vi "Convert_ERDs_ARG.vi"(0 "New Header?":bool, 2 "ERD Name":string[](array[string]), 5 "All_Bundled_Data_Brass":T1, 7 "Array":T8[](array[typedef]) {"ERD Number" format="%.0x"}, 11 "Error In":errorcluster) -> (6 "All_ERD_Data_Bundled_Brass":T1, 15 "Error Out":errorcluster)   [LabVIEW 2023]
doc: "This VI parses the data from ERDs in correct format, units, etc. It handles all hex to dec conversions, hex to enum, and hex to boolean conversions.\n\nIf Raw Data from ERD is blank string, then it will output values from shift register."
uses:
  Common/LabVIEW GEA2 Toolkit/GEA3/type defs/ERD Read Data Out.ctl
  Type defs/All_Bundled_Data_ARG.ctl
  Common/type defs/Version.ctl
  Common/type defs/CSV_File_String_Arrays.ctl
  Common/type defs/Fault Table Array.ctl
  Common/type defs/Fault_Table_Info.ctl
  Type defs/ERD_Always_Show_ARG.ctl
  Common/type defs/BootloaderVersion.ctl
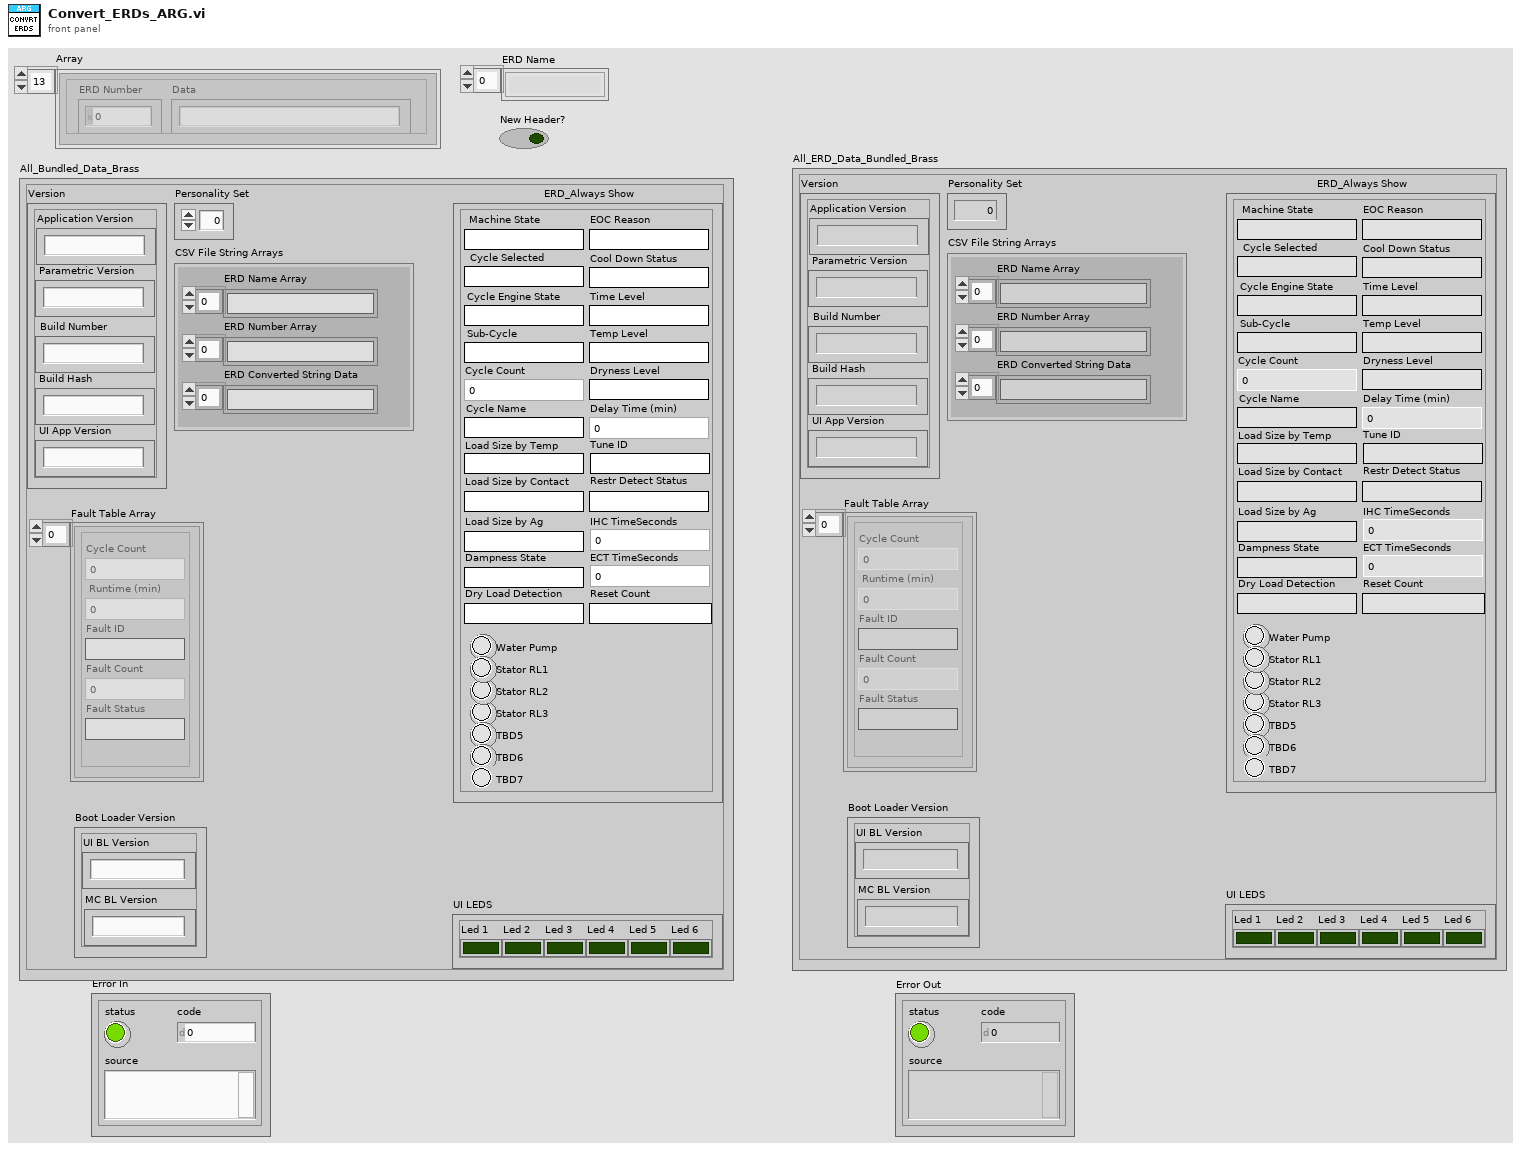
[diagram p1: front panel]
types:
  T1 = typedef "All_Bundled_Data_ARG.ctl" = cluster{"Version":T2, "Personality Set":u8, "CSV File String Arrays":T3, "Fault Table Array ":T4, "ERD_Always Show":T6, "UI LEDS":cluster{"Led 1":bool, "Led 2":bool, "Led 3":bool, "Led 4":bool, "Led 5":bool, "Led 6":bool}, "Boot Loader Version":T7}
  T2 = typedef "Version.ctl" = cluster{"Build Number":string, "Build Hash ":string, "Application Version":string, "Parametric Version":string, "UI App Version":string}
  T3 = typedef "CSV_File_String_Arrays.ctl" = cluster{"ERD Number Array":string[], "ERD Name Array":string[], "ERD Converted String Data":string[]}
  T4 = typedef "Fault Table Array.ctl" = T5[]
  T5 = typedef "Fault_Table_Info.ctl" = cluster{"Cycle Count":u32, " Runtime (min) ":u32, "Fault Status":string, "Fault ID":string, "Fault Count":u16}
  T6 = typedef "ERD_Always_Show_ARG.ctl" = cluster{"Machine State":string, "Cycle Selected":string, "Cycle Engine State":string, "Cycle Count":u32, "Temp Level":string, "Dryness Level":string, "Time Level":string, "Delay Time (min)":u16, "Sub-Cycle":string, "Cycle Name":string, "Tune ID":string, "Restr Detect Status":string, "Load Size by Contact":string, "Load Size by Temp":string, "EOC Reason":string, "Reset Count":string, "Dampness State":string, "Stator RL3":bool, "TBD5":bool, "TBD6":bool, "Water Pump":bool, "Stator RL2":bool, "Cool Down Status":string, "TBD7":bool, "Stator RL1":bool, "IHC TimeSeconds":u32, "ECT TimeSeconds ":u32, "Load Size by Ag":string, "Dry Load Detection":string}
  T7 = typedef "BootloaderVersion.ctl" = cluster{"UI BL Version":string, "MC BL Version":string}
  T8 = typedef "ERD Read Data Out.ctl" = cluster{"ERD Number":u16, "Data":string}
  T9 = cluster{"Led 1":bool, "Led 2":bool, "Led 3":bool, "Led 4":bool, "Led 5":bool, "Led 6":bool}
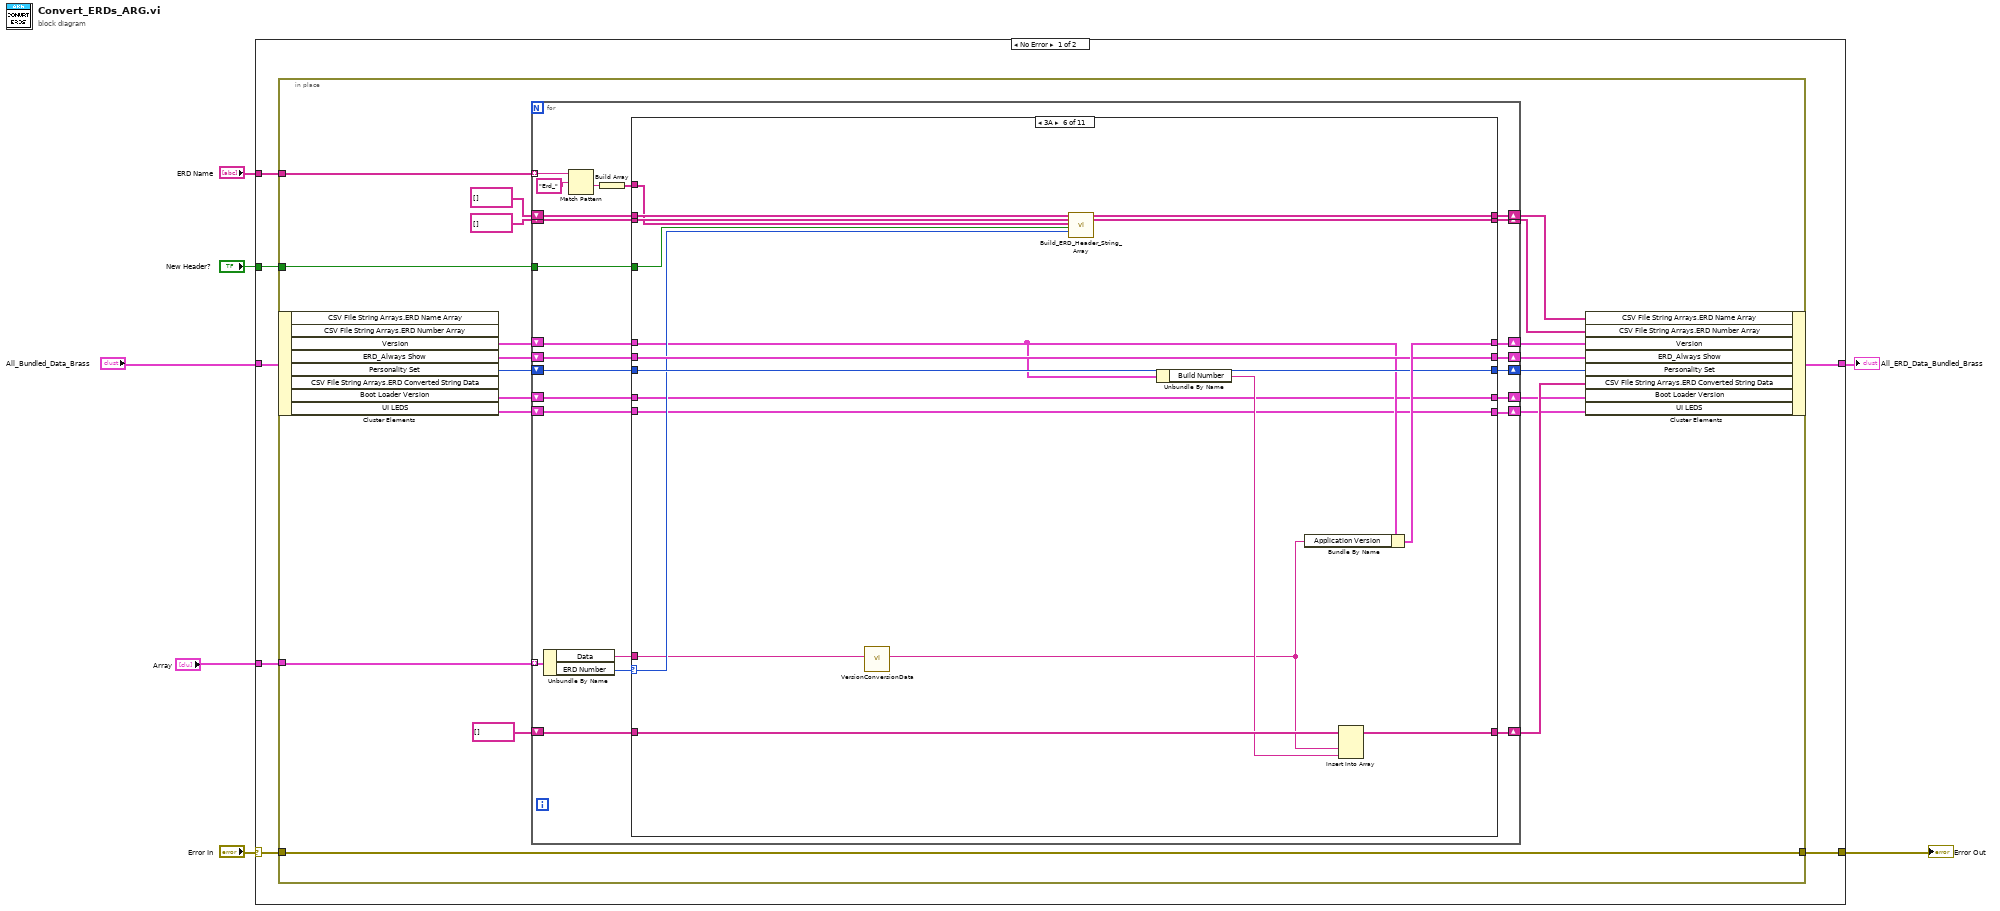
[diagram p0: block diagram]
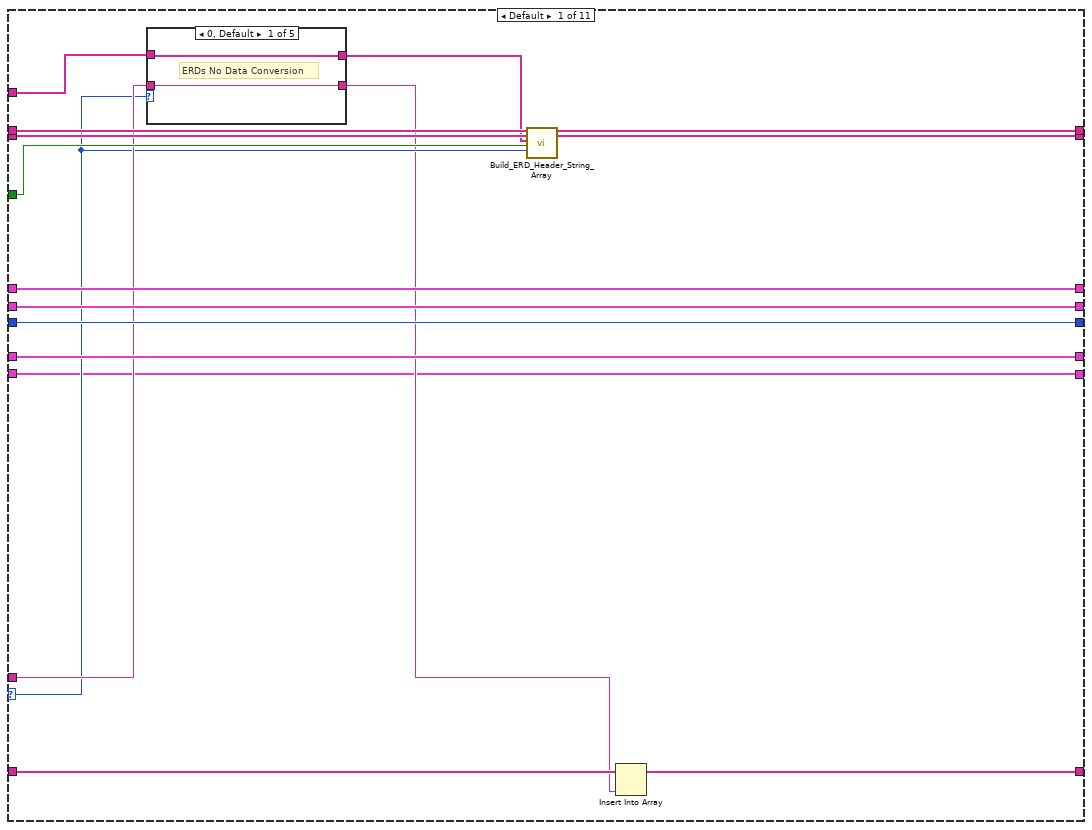
[diagram p2: hidden frame]
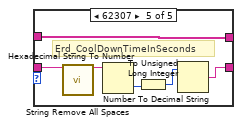
[diagram p6: hidden frame]
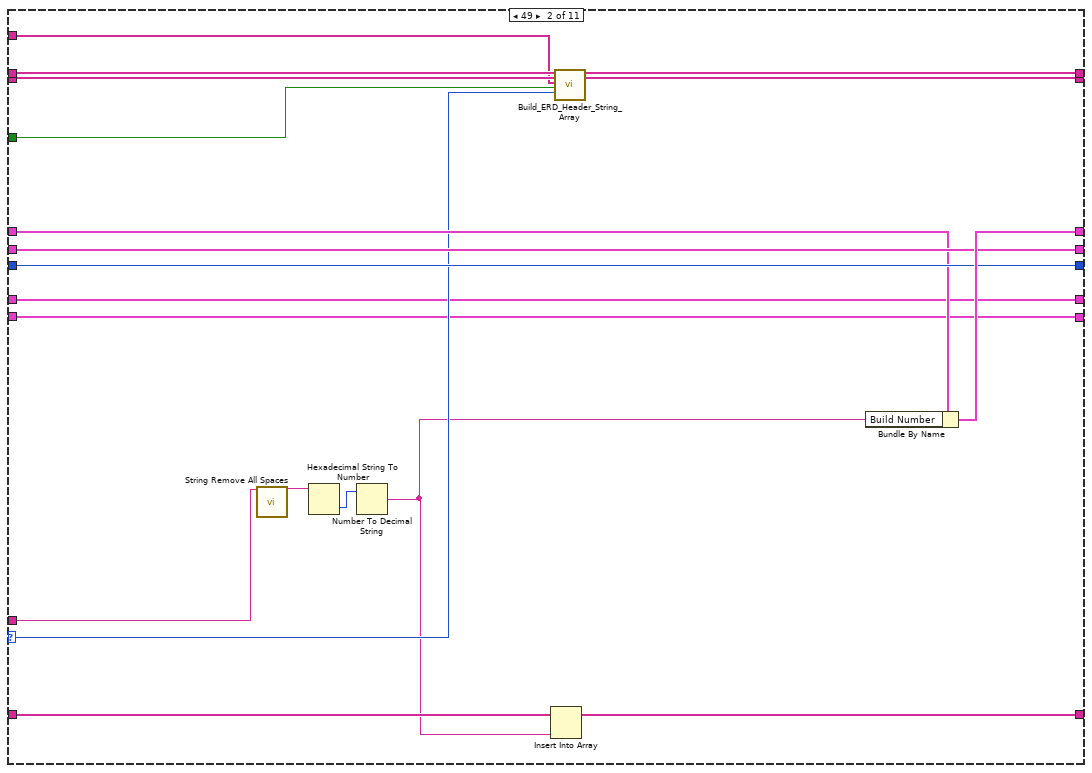
[diagram p7: hidden frame]
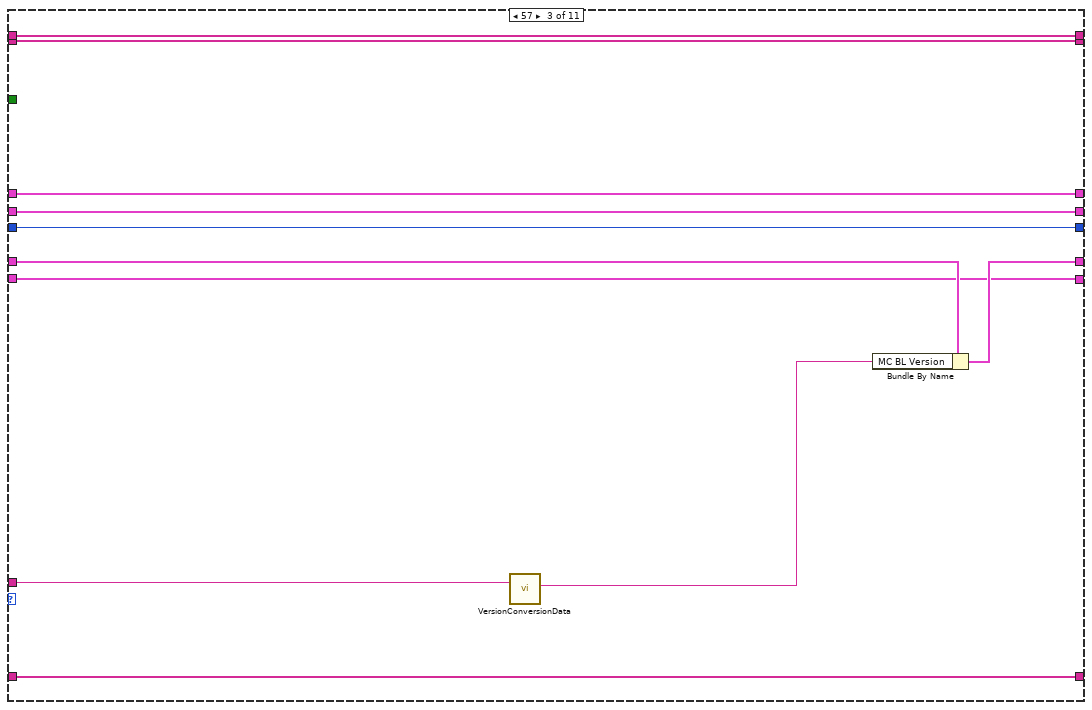
[diagram p8: hidden frame]
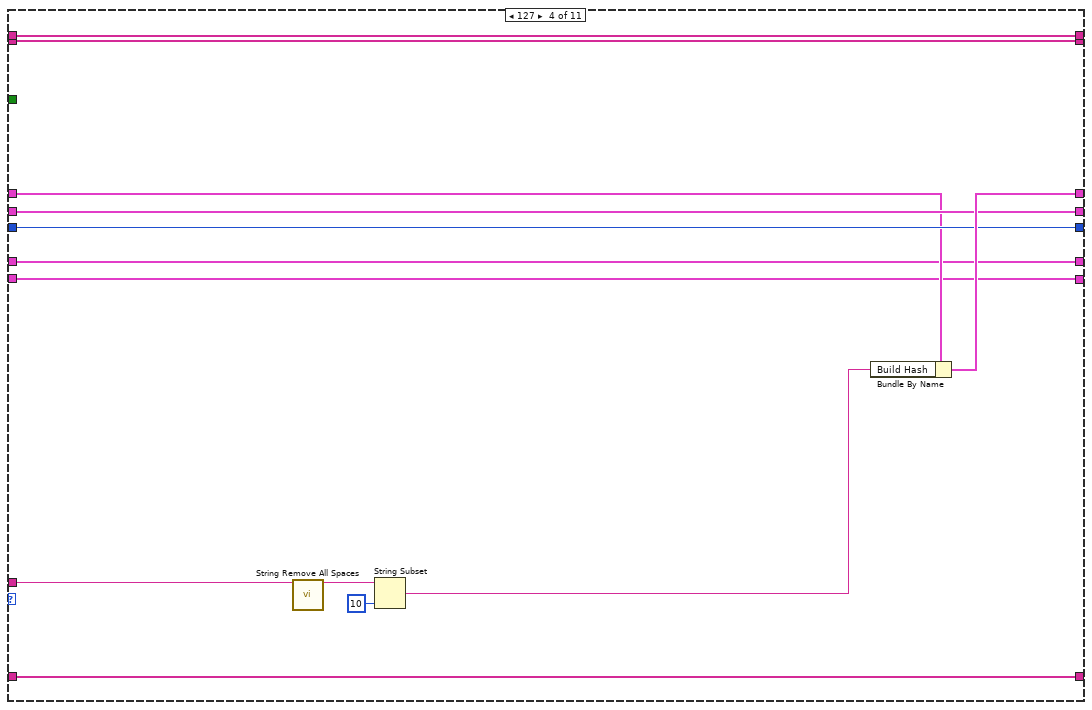
[diagram p9: hidden frame]
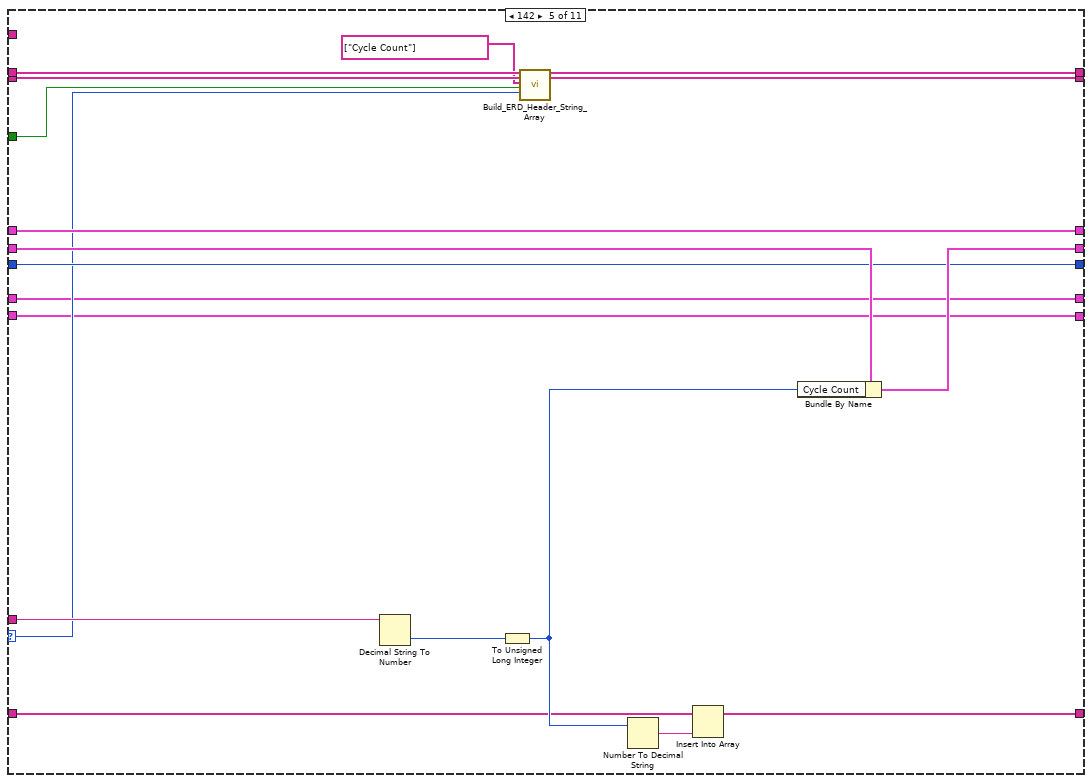
[diagram p10: hidden frame]
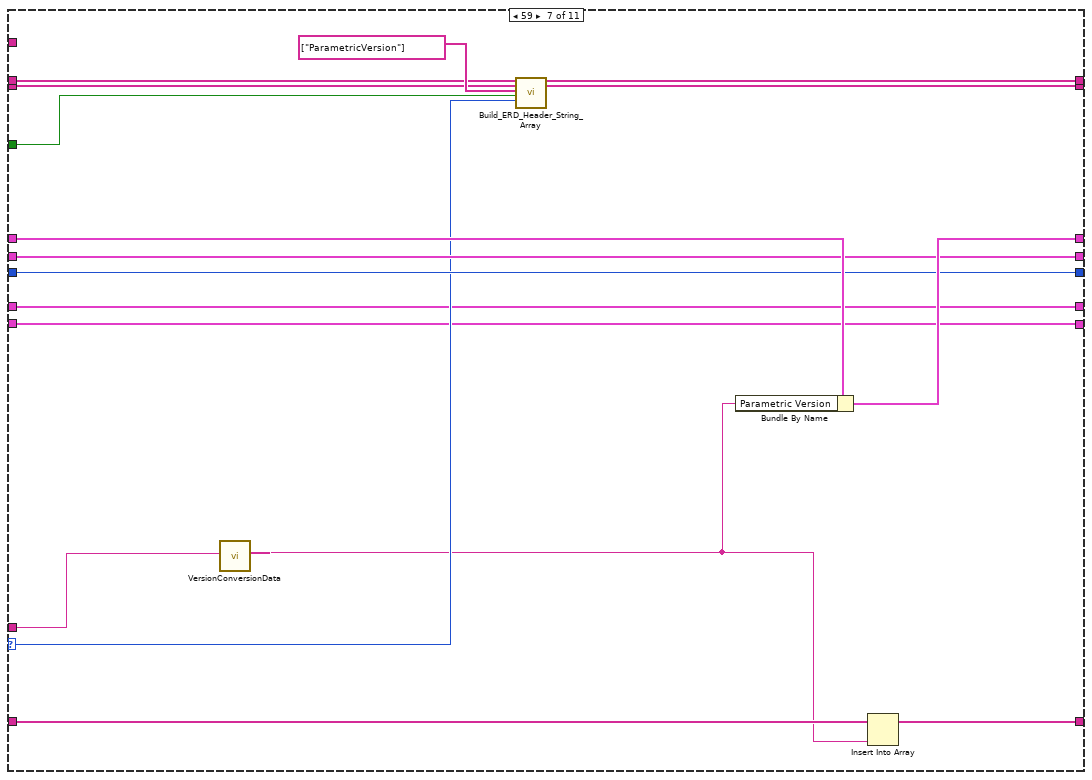
[diagram p11: hidden frame]
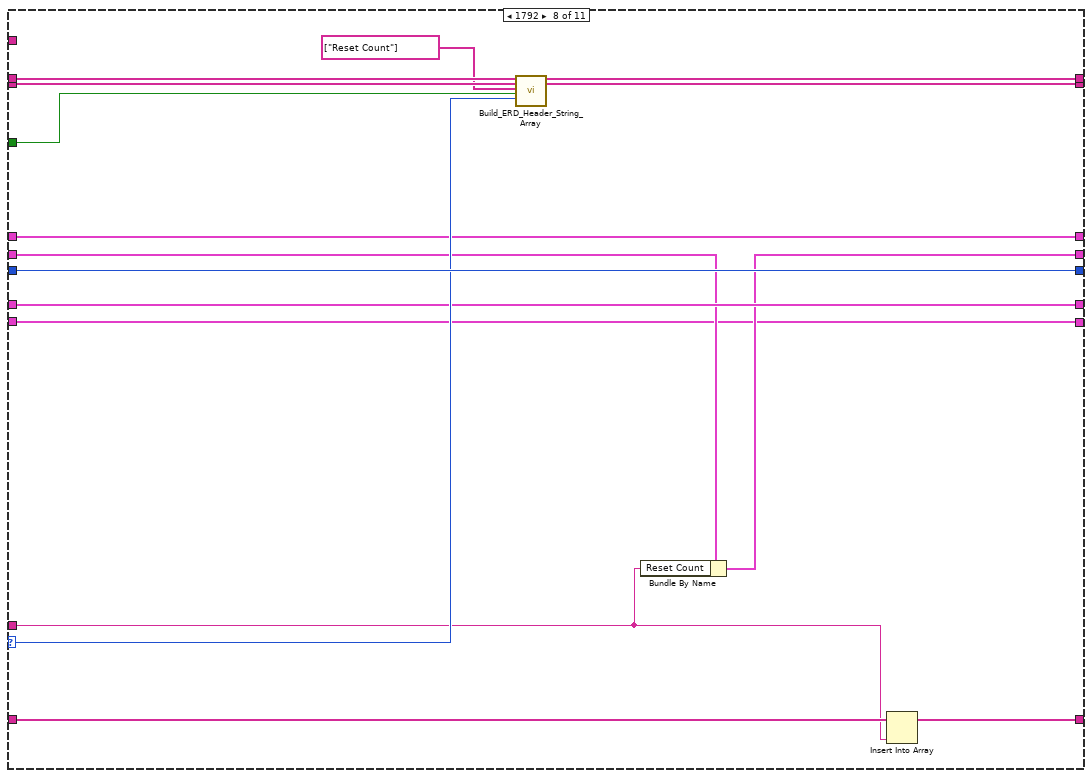
[diagram p12: hidden frame]
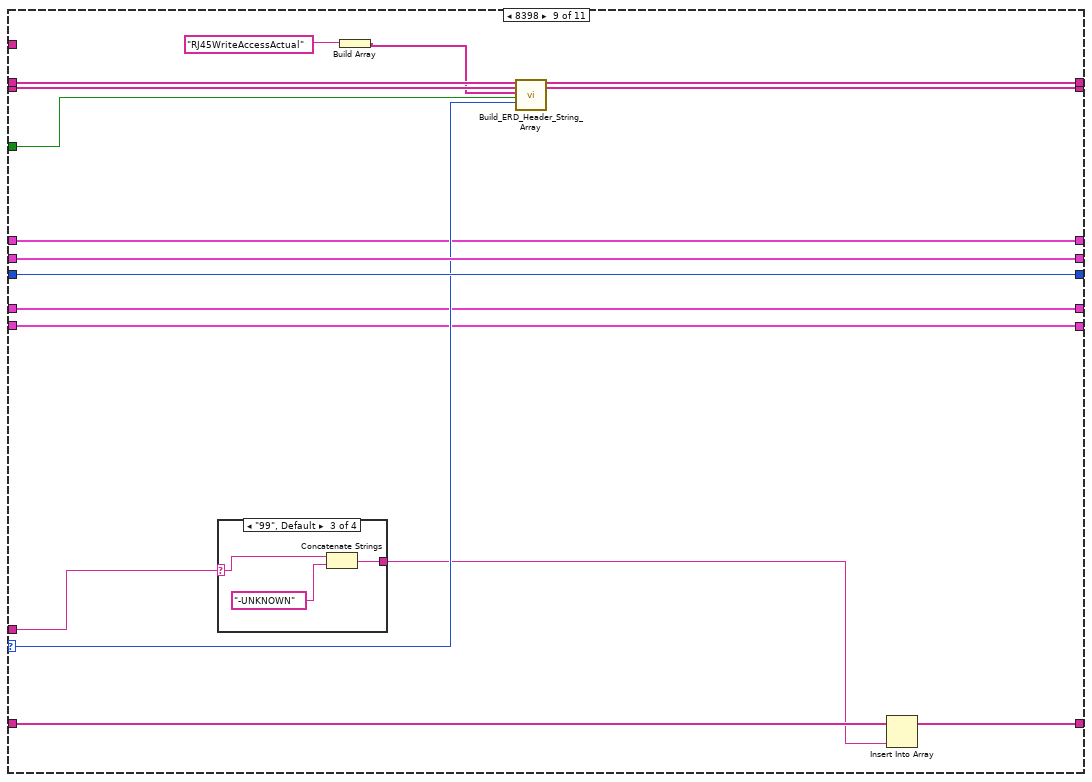
[diagram p13: hidden frame]
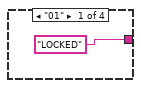
[diagram p14: hidden frame]
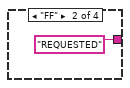
[diagram p15: hidden frame]
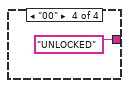
[diagram p16: hidden frame]
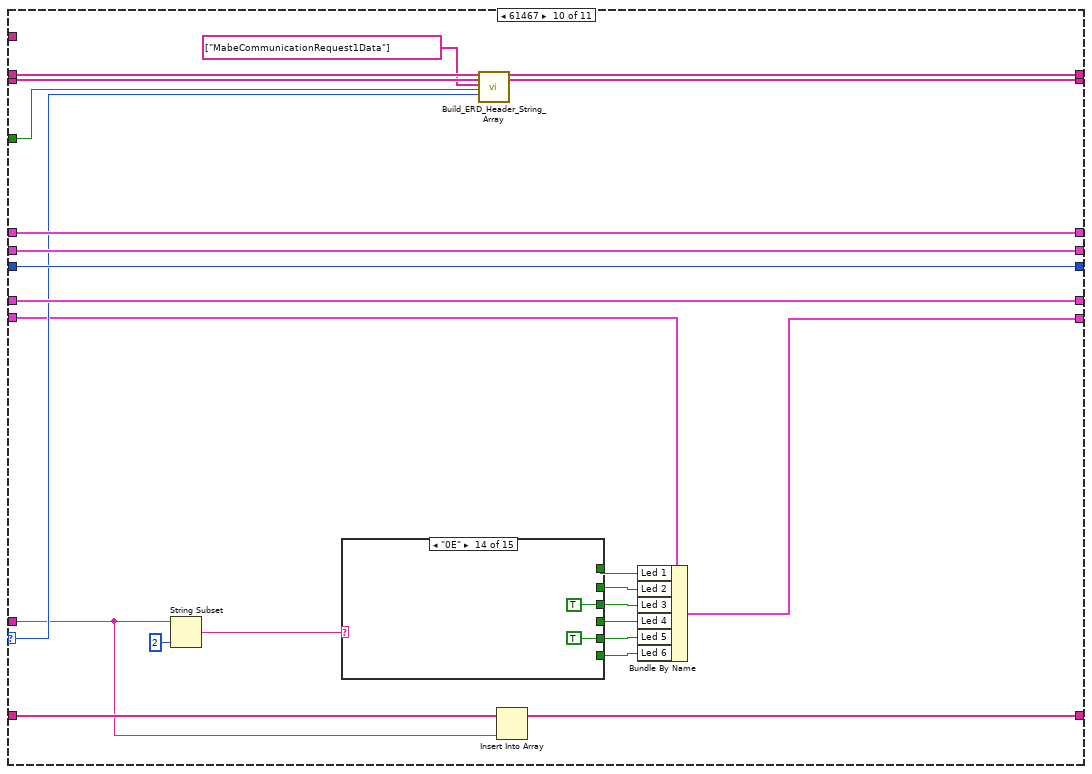
[diagram p17: hidden frame]
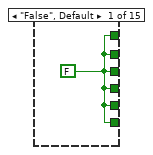
[diagram p18: hidden frame]
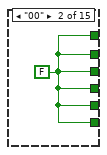
[diagram p19: hidden frame]
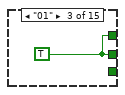
[diagram p20: hidden frame]
diagram:
  n1 = case shown="No Error" "Error In" {
    selector: "Error In" -> [w11 w291]
    tunnel: "Array" -> [w14 _]
    tunnel: [w12 w290] -> w5
    tunnel: "All_Bundled_Data_Brass" -> [w13 w289]
    tunnel: [w10 w289] -> w1
    tunnel: "New Header?" -> [w9 _]
    tunnel: "ERD Name" -> [w8 _]
    frame No Error {
      n2 = in-place {
        in-place-border: w14 -> [w18]
        in-place-border: [w17] -> w12
        in-place-border: w11 -> [w17]
        in-place-border: w9 -> [w27]
        in-place-border: w8 -> [w19]
        n3 = in-place-cluster #1(w13) -> ("Version"=w33:T2, "ERD_Always Show"=w34:T6, "Personality Set"=w30:u8, "Boot Loader Version"=w21:T7, "UI LEDS"=w16:T9)  [unwired: 3 out]
        n4 = for {
          shift-right: [w57] -> w31
          shift-left: w34 -> [w56]
          shift-right: [w54] -> w32
          shift-left: w33 -> [w55]
          shift-right: [w51] -> w29
          shift-left: w30 -> [w52]
          shift-right: [w49] -> w22
          shift-left: string[] [] ("ERD String Data") -> [w50]
          tunnel: w27 -> [w48]
          shift-right: [w44] -> w23
          shift-left: string[] [] ("ERD String Data") -> [w47]
          shift-right: [w45] -> w24
          shift-left: string[] [] ("ERD String Data") -> [w46]
          shift-right: [w36] -> w20
          shift-left: w21 -> [w43]
          tunnel: w19 -> [w42] mode=indexing
          tunnel: w18 -> [w38] mode=indexing
          shift-right: [w35] -> w15
          shift-left: w16 -> [w37]
          n5 = Unbundle By Name(w38) -> ("Data"=w58:string, "ERD Number"=w53:u16)
          n6 = Match Pattern(string=w42, regular expression="Erd_") -> (after substring=w39:string)  [unwired: 1 in, 3 out]
          n7 = Build Array(w39) -> (w40:string[])
          n8 = case shown="3A" w53 {
            selector: w53 -> [w61 w100 _ _ w140 w161 w174 w194 w210 w244 w274]
            tunnel: w58 -> [w62 w95 w111 w126 w151 w155 w172 w190 w207 w230 w271]
            tunnel: [w75 w107 w119 w131 w149 w168 w184 w189 w219 w249 w283] -> w57
            tunnel: w56 -> [w75 w107 w119 w131 w150 w168 w184 w191 w219 w249 w283]
            tunnel: w55 -> [w74 w105 w112 w127 w148 w160 w186 w192 w206 w248 w270]
            tunnel: [w74 w108 w112 w132 w148 w169 w185 w192 w206 w248 w270] -> w54
            tunnel: w52 -> [w73 w106 w118 w130 w147 w167 w183 w202 w218 w247 w282]
            tunnel: [w73 w106 w118 w130 w147 w167 w183 w202 w218 w247 w282] -> w51
            tunnel: w50 -> [w71 w104 w115 w122 w145 w156 w178 w198 w214 w227 w278]
            tunnel: [w67 w103 w115 w122 w143 w163 w176 w196 w212 w242 w276] -> w49
            tunnel: w48 -> [w69 w99 _ _ w141 w162 w175 w195 w211 w245 w275]
            tunnel: w47 -> [w70 w102 w116 w128 w146 w157 w179 w199 w215 w228 w279]
            tunnel: w46 -> [w65 w97 w117 w129 w136 w166 w182 w201 w217 w231 w281]
            tunnel: [w66 w96 w117 w129 w135 w165 w181 w200 w216 w229 w280] -> w45
            tunnel: [w68 w101 w116 w128 w144 w164 w177 w197 w213 w243 w277] -> w44
            tunnel: w43 -> [w72 w98 w114 w121 w134 w158 w173 w193 w209 w246 w273]
            tunnel: [w72 w98 w113 w121 w134 w158 w173 w193 w209 w246 w273] -> w36
            tunnel: w40 -> [w63 w90 _ _ _ w152 _ _ _ _ _]
            tunnel: w37 -> [w59 w91 w109 w120 w133 w153 w170 w188 w203 w240 w267]
            tunnel: [w59 w91 w109 w120 w133 w153 w170 w188 w203 w239 w267] -> w35
            frame Default {
              n9 = case shown="0, Default" w61 {
                tunnel: [w76 w79 w81 w83 w89] -> w64
                tunnel: w63 -> [w76 w79 w81 w83 w89]
                tunnel: w62 -> [w77 w78 w80 w82 w86]
                tunnel: [w77 w78 w80 w82 w84] -> w60
                frame 0, Default {
                  # "ERDs No Data Conversion"
                }
                frame 65423 {
                  # "Consumer Error Mode"
                }
                frame 55 {
                  # "ServiceModeState"
                }
                frame 61811 {
                  # "WiFiCommissioningOption"
                }
                frame 62307 {
                  # "Erd_CoolDownTimeInSeconds"
                  n10 = call "String Remove All Spaces.vi"("Input String"=w86) -> ("Spaces Removed"=w87:string)  [unwired: 13 in, 1 out]
                  n11 = Hexadecimal String To Number(string=w87) -> (number=w88:u32)  [unwired: 2 in, 1 out]
                  n12 = To Unsigned Long Integer(number=w88) -> (unsigned 32bit integer=w85:u32)
                  n13 = Number To Decimal String(number=w85) -> (decimal integer string=w84:string)  [unwired: 1 in]
                }
              }
              n14 = call "Build_ERD_Header_String_Array.vi"("ERD Name Array In"=w70, "ERD Number Array In"=w71, "ERD Name List"=w64, "New Header?"=w69, "ERD Number"=w61) -> ("ERD Name Array Out"=w68:string[], "ERD Number Array Out"=w67:string[])  [unwired: 13 in]
              n15 = Insert Into Array(array=w65, new element=w60) -> (w66:string[])  [unwired: 1 in]
            }
            frame 49 {
              n16 = call "String Remove All Spaces.vi"("Input String"=w95) -> ("Spaces Removed"=w94:string)  [unwired: 13 in, 1 out]
              n17 = Hexadecimal String To Number(string=w94) -> (number=w92:u32)  [unwired: 2 in, 1 out]
              n18 = Number To Decimal String(number=w92) -> (decimal integer string=w93:string)  [unwired: 1 in]
              n19 = Insert Into Array(array=w97, new element=w93) -> (w96:string[])  [unwired: 1 in]
              n20 = call "Build_ERD_Header_String_Array.vi"("ERD Name Array In"=w102, "ERD Number Array In"=w104, "ERD Name List"=w90, "New Header?"=w99, "ERD Number"=w100) -> ("ERD Name Array Out"=w101:string[], "ERD Number Array Out"=w103:string[])  [unwired: 13 in]
              n21 = Bundle By Name(cluster=w105, "Build Number"=w93) -> (w108:T2)
            }
            frame 57 {
              n22 = call "VersionConversionData.vi"("Version In"=w111) -> ("Version Out"=w110:string)  [unwired: 9 in, 1 out]
              n23 = Bundle By Name(cluster=w114, "MC BL Version"=w110) -> (w113:T7)
            }
            frame 127 {
              n24 = call "String Remove All Spaces.vi"("Input String"=w126) -> ("Spaces Removed"=w125:string)  [unwired: 13 in, 1 out]
              n25 = String Subset(string=w125, length (rest)=10 ("length (rest)")) -> (substring=w123:string)  [unwired: 1 in]
              n26 = Bundle By Name(cluster=w127, "Build Hash"=w123) -> (w132:T2)
            }
            frame 142 {
              n27 = Decimal String To Number(string=w151) -> (number=w138:i32)  [unwired: 2 in, 1 out]
              n28 = To Unsigned Long Integer(number=w138) -> (unsigned 32bit integer=w137:u32)
              n29 = call "Build_ERD_Header_String_Array.vi"("ERD Name Array In"=w146, "ERD Number Array In"=w145, "ERD Name List"=string[] ["Cycle Count"], "New Header?"=w141, "ERD Number"=w140) -> ("ERD Name Array Out"=w144:string[], "ERD Number Array Out"=w143:string[])  [unwired: 13 in]
              n30 = Number To Decimal String(number=w137) -> (decimal integer string=w139:string)  [unwired: 1 in]
              n31 = Insert Into Array(array=w136, new element=w139) -> (w135:string[])  [unwired: 1 in]
              n32 = Bundle By Name(cluster=w150, "Cycle Count"=w137) -> (w149:T6)
            }
            frame 58 {
              n33 = call "VersionConversionData.vi"("Version In"=w155) -> ("Version Out"=w154:string)  [unwired: 9 in, 1 out]
              n34 = call "Build_ERD_Header_String_Array.vi"("ERD Name Array In"=w157, "ERD Number Array In"=w156, "ERD Name List"=w152, "New Header?"=w162, "ERD Number"=w161) -> ("ERD Name Array Out"=w164:string[], "ERD Number Array Out"=w163:string[])  [unwired: 13 in]
              n35 = Unbundle By Name(w160) -> ("Build Number"=w159:string)
              n36 = Bundle By Name(cluster=w160, "Application Version"=w154) -> (w169:T2)
              n37 = Insert Into Array(array=w166, new element #1=w154, new element #2=w159) -> (w165:string[])  [unwired: 1 in]
            }
            frame 59 {
              n38 = call "VersionConversionData.vi"("Version In"=w172) -> ("Version Out"=w171:string)  [unwired: 9 in, 1 out]
              n39 = call "Build_ERD_Header_String_Array.vi"("ERD Name Array In"=w179, "ERD Number Array In"=w178, "ERD Name List"=string[] ["ParametricVersion"], "New Header?"=w175, "ERD Number"=w174) -> ("ERD Name Array Out"=w177:string[], "ERD Number Array Out"=w176:string[])  [unwired: 13 in]
              n40 = Bundle By Name(cluster=w186, "Parametric Version"=w171) -> (w185:T2)
              n41 = Insert Into Array(array=w182, new element=w171) -> (w181:string[])  [unwired: 1 in]
            }
            frame 1792 {
              n42 = call "Build_ERD_Header_String_Array.vi"("ERD Name Array In"=w199, "ERD Number Array In"=w198, "ERD Name List"=string[] ["Reset Count"], "New Header?"=w195, "ERD Number"=w194) -> ("ERD Name Array Out"=w197:string[], "ERD Number Array Out"=w196:string[])  [unwired: 13 in]
              n43 = Bundle By Name(cluster=w191, "Reset Count"=w190) -> (w189:T6)
              n44 = Insert Into Array(array=w201, new element=w190) -> (w200:string[])  [unwired: 1 in]
            }
            frame 8398 {
              n45 = case shown="\"99\", Default" w207 {
                selector: w207 -> [_ _ w224 _]
                tunnel: ["LOCKED" ("Write Access") "REQUESTED" ("Write Access") w222 "UNLOCKED" ("Write Access")] -> w204
                frame "01" {
                }
                frame "FF" {
                }
                frame "99", Default {
                  n46 = Concatenate Strings(w224, "-UNKNOWN" ("Write Access")) -> (w222:string)
                }
                frame "00" {
                }
              }
              n47 = Build Array("RJ45WriteAccessActual" ("String")) -> (w208:string[])
              n48 = call "Build_ERD_Header_String_Array.vi"("ERD Name Array In"=w215, "ERD Number Array In"=w214, "ERD Name List"=w208, "New Header?"=w211, "ERD Number"=w210) -> ("ERD Name Array Out"=w213:string[], "ERD Number Array Out"=w212:string[])  [unwired: 13 in]
              n49 = Insert Into Array(array=w217, new element=w204) -> (w216:string[])  [unwired: 1 in]
            }
            frame 61467 {
              n50 = String Subset(string=w230, length (rest)=2 ("length (rest)")) -> (substring=w241:string)  [unwired: 1 in]
              n51 = case shown="\"0E\"" w241 {
                tunnel: [w250 w251 w252 w253 w254 w255 w256 TRUE _ _ _ _ _ _ _] -> w238
                tunnel: [w250 w251 w252 w253 w254 w255 w256 _ TRUE _ _ _ _ _ TRUE] -> w237
                tunnel: [w250 w251 _ w253 w254 w255 w256 _ _ TRUE _ _ _ TRUE _] -> w236
                tunnel: [w250 w251 _ _ w254 w255 w256 _ _ _ TRUE _ _ _ _] -> w235
                tunnel: [w250 w251 _ _ _ w255 w256 _ _ _ _ TRUE _ TRUE _] -> w234
                tunnel: [w250 w251 _ _ _ _ w256 _ _ _ _ _ TRUE _ TRUE] -> w233
                frame "False", Default {
                  w250 = FALSE
                }
                frame "00" {
                  w251 = FALSE
                }
                frame "01" {
                  w252 = TRUE
                }
                frame "02" {
                  w253 = TRUE
                }
                frame "03" {
                  w254 = TRUE
                }
                frame "04" {
                  w255 = TRUE
                }
                frame "05" {
                  w256 = TRUE
                }
                frame "07" {
                }
                frame "08" {
                }
                frame "09" {
                }
                frame "0A" {
                }
                frame "0B" {
                }
                frame "0C" {
                }
                frame "0E" {
                }
                frame "0F" {
                }
              }
              n52 = call "Build_ERD_Header_String_Array.vi"("ERD Name Array In"=w228, "ERD Number Array In"=w227, "ERD Name List"=string[] ["MabeCommunicationRequest1Data"], "New Header?"=w245, "ERD Number"=w244) -> ("ERD Name Array Out"=w243:string[], "ERD Number Array Out"=w242:string[])  [unwired: 13 in]
              n53 = Insert Into Array(array=w231, new element=w230) -> (w229:string[])  [unwired: 1 in]
              n54 = Bundle By Name(cluster=w240, "Led 1"=w238, "Led 2"=w237, "Led 3"=w236, "Led 4"=w235, "Led 5"=w234, "Led 6"=w233) -> (w239:T9)
            }
            frame 65522 {
              n55 = case shown="\"00\"" w271 {
                selector: w271 -> [_ w287 _]
                tunnel: ["LOCKED" ("Write Access") w285 "UNLOCKED" ("Write Access")] -> w268
                frame "01" {
                }
                frame "99", Default {
                  n56 = Concatenate Strings(w287, "-UNKNOWN" ("Write Access")) -> (w285:string)
                }
                frame "00" {
                }
              }
              n57 = Build Array("Rj45LockedAtLeastOnce" ("String")) -> (w272:string[])
              n58 = call "Build_ERD_Header_String_Array.vi"("ERD Name Array In"=w279, "ERD Number Array In"=w278, "ERD Name List"=w272, "New Header?"=w275, "ERD Number"=w274) -> ("ERD Name Array Out"=w277:string[], "ERD Number Array Out"=w276:string[])  [unwired: 13 in]
              n59 = Insert Into Array(array=w281, new element=w268) -> (w280:string[])  [unwired: 1 in]
            }
          }
        }
        n60 = in-place-cluster #1("CSV File String Arrays.ERD Name Array"=w23, "CSV File String Arrays.ERD Number Array"=w22, "Version"=w32, "ERD_Always Show"=w31, "Personality Set"=w29, "CSV File String Arrays.ERD Converted String Data"=w24, "Boot Loader Version"=w20, "UI LEDS"=w15) -> (w10:T1)
      }
    }
    frame Error {
      n61 = Unbundle By Name(w291) -> ("code"=w295:i32, "status"=w296:bool, "source"=w293:string)
      n62 = Equal?(x=w295, y=-5006) -> (x = y?=w299:bool)
      n63 = case shown="True" w299 {
        tunnel: [w303 FALSE] -> w297
        tunnel: w296 -> [w303 _]
        tunnel: w295 -> [w302 w305]
        tunnel: [w302 w305] -> w294
        tunnel: [w301 w304] -> w292
        tunnel: w293 -> [w301 w304]
        frame False {
        }
        frame True {
        }
      }
      n64 = Bundle By Name(cluster=errorcluster {"status"=FALSE, "code"=0, "source"=""} ("error constant"), "status"=w297, "code"=w294, "source"=w292) -> (w290:errorcluster)
    }
  }
  "Error Out" <- w5
  "All_ERD_Data_Bundled_Brass" <- w1
